vi "HEWH Filter All Temps.vi"(6 "Good Scan?":bool, 8 "error in (no error)":errorcluster, 11 "Pressure Adjusted in":T1) -> (0 "error out":errorcluster, 2 "TC Tree Array":dbl[](array[numeric]), 3 "Pressure Adjusted out":T1)   [LabVIEW 2023]
uses:
  Type Definitions/HEWH MW100 Data Cluster.ctl
  <vilib>/Analysis/NI_AALBase.lvlib
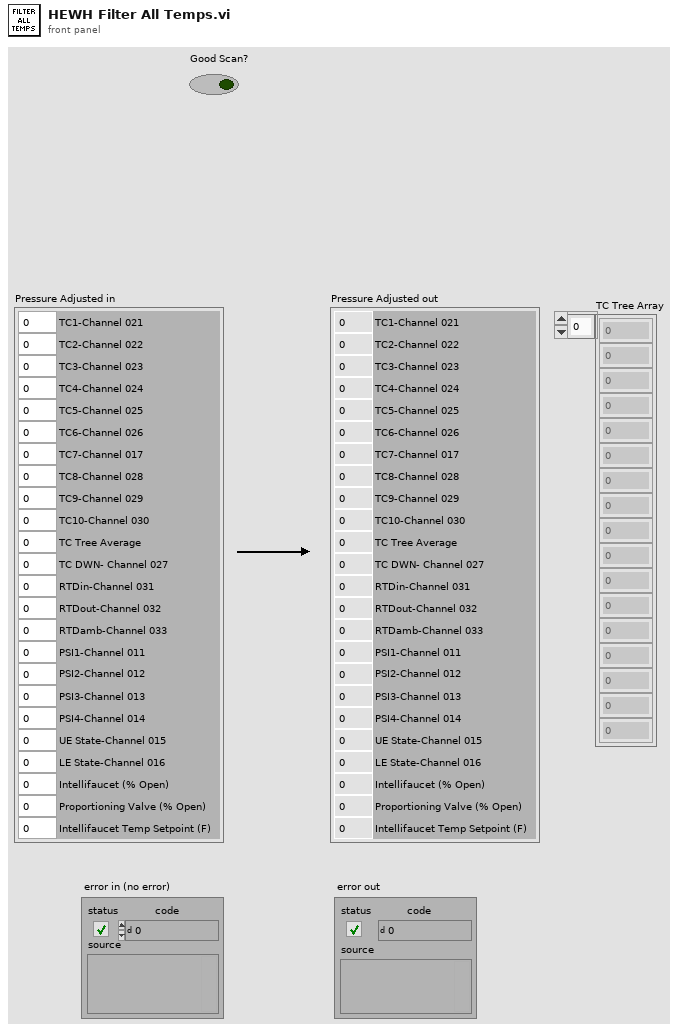
[diagram p1: front panel]
types:
  T1 = typedef "HEWH MW100 Data Cluster.ctl" = cluster{"TC1-Channel 021":dbl, "TC2-Channel 022":dbl, "TC3-Channel 023":dbl, "TC4-Channel 024":dbl, "TC5-Channel 025":dbl, "TC6-Channel 026":dbl, "TC7-Channel 017":dbl, "TC8-Channel 028":dbl, "TC9-Channel 029":dbl, "TC10-Channel 030":dbl, "TC Tree Average":dbl, "TC DWN- Channel 027":dbl, "RTDin-Channel 031":dbl, "RTDout-Channel 032":dbl, "RTDamb-Channel 033":dbl, "PSI1-Channel 011":dbl, "PSI2-Channel 012":dbl, "PSI3-Channel 013":dbl, "PSI4-Channel 014":dbl, "UE State-Channel 015":dbl, "LE State-Channel 016":dbl, "Intellifaucet (% Open)":dbl, "Proportioning Valve (% Open)":dbl, "Intellifaucet Temp Setpoint (F)":dbl}
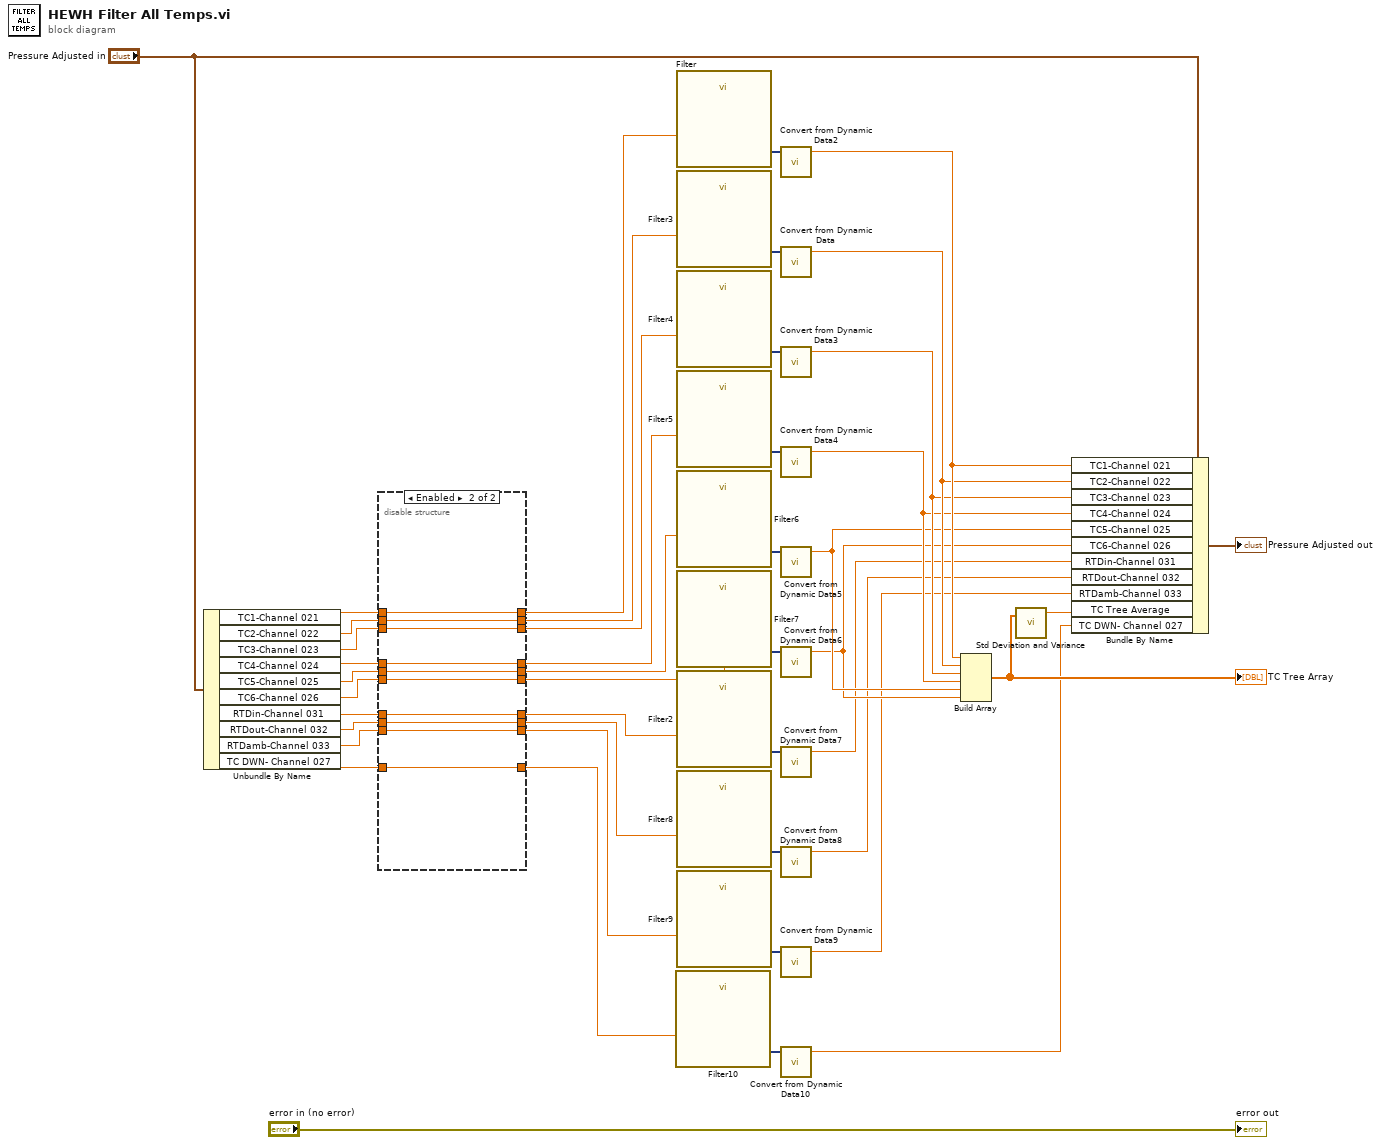
[diagram p0: block diagram]
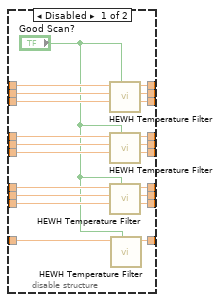
[diagram p2: hidden frame]
diagram:
  n1 = Unbundle By Name("Pressure Adjusted in") -> ("TC1-Channel 021"=w42:dbl, "TC2-Channel 022"=w41:dbl, "TC3-Channel 023"=w40:dbl, "TC4-Channel 024"=w39:dbl, "TC5-Channel 025"=w38:dbl, "TC6-Channel 026"=w37:dbl, "RTDin-Channel 031"=w36:dbl, "RTDout-Channel 032"=w35:dbl, "RTDamb-Channel 033"=w34:dbl, "TC DWN- Channel 027"=w5:dbl)
  n2 = disable-structure shown="Enabled" {
    disable-tunnel: w42 -> [w66 w76]
    disable-tunnel: w41 -> [w65 w75]
    disable-tunnel: w40 -> [w64 w74]
    disable-tunnel: w39 -> [w63 w73]
    disable-tunnel: w38 -> [w62 w72]
    disable-tunnel: w37 -> [w61 w71]
    disable-tunnel: w36 -> [w60 w70]
    disable-tunnel: w35 -> [w59 w69]
    disable-tunnel: w34 -> [w58 w68]
    disable-tunnel: [w57 w76] -> w33
    disable-tunnel: [w56 w74] -> w32
    disable-tunnel: [w55 w73] -> w31
    disable-tunnel: [w54 w72] -> w30
    disable-tunnel: [w53 w71] -> w29
    disable-tunnel: [w52 w70] -> w28
    disable-tunnel: [w51 w69] -> w27
    disable-tunnel: [w50 w68] -> w26
    disable-tunnel: [w49 w75] -> w14
    disable-tunnel: w5 -> [w48 w67]
    disable-tunnel: [w46 w67] -> w2
    frame Disabled {
      n3 = call "HEWH Temperature Filter.vi"("Good Scan?"="Good Scan?", "Temperature 3 Inlet"=w64, "Temperature 2 Inlet"=w65, "Temperature 1 Inlet"=w66) -> ("Temperature 3 Outlet"=w56:dbl, "Temperature 2 Outlet"=w49:dbl, "Temperature 1 Outlet"=w57:dbl)  [unwired: 5 in]
      n4 = call "HEWH Temperature Filter.vi"("Good Scan?"="Good Scan?", "Temperature 3 Inlet"=w61, "Temperature 2 Inlet"=w62, "Temperature 1 Inlet"=w63) -> ("Temperature 3 Outlet"=w53:dbl, "Temperature 2 Outlet"=w54:dbl, "Temperature 1 Outlet"=w55:dbl)  [unwired: 5 in]
      n5 = call "HEWH Temperature Filter.vi"("Good Scan?"="Good Scan?", "Temperature 3 Inlet"=w58, "Temperature 2 Inlet"=w59, "Temperature 1 Inlet"=w60) -> ("Temperature 3 Outlet"=w50:dbl, "Temperature 2 Outlet"=w51:dbl, "Temperature 1 Outlet"=w52:dbl)  [unwired: 5 in]
      n6 = call "HEWH Temperature Filter.vi"("Good Scan?"="Good Scan?", "Temperature 1 Inlet"=w48) -> ("Temperature 1 Outlet"=w46:dbl)  [unwired: 7 in, 2 out]
    }
    frame Enabled {
    }
  }
  n7 = call "Filter10"("Signal"=w2) -> ("Filtered Signal"=w4:dynamicdata)  [unwired: 9 in, 1 out]
  n8 = call "Filter"("Signal"=w33) -> ("Filtered Signal"=w25:dynamicdata)  [unwired: 9 in, 1 out]
  n9 = call "Filter3"("Signal"=w14) -> ("Filtered Signal"=w24:dynamicdata)  [unwired: 9 in, 1 out]
  n10 = call "Filter4"("Signal"=w32) -> ("Filtered Signal"=w23:dynamicdata)  [unwired: 9 in, 1 out]
  n11 = call "Filter5"("Signal"=w31) -> ("Filtered Signal"=w22:dynamicdata)  [unwired: 9 in, 1 out]
  n12 = call "Filter6"("Signal"=w30) -> ("Filtered Signal"=w21:dynamicdata)  [unwired: 9 in, 1 out]
  n13 = call "Filter7"("Signal"=w29) -> ("Filtered Signal"=w20:dynamicdata)  [unwired: 9 in, 1 out]
  n14 = call "Filter2"("Signal"=w28) -> ("Filtered Signal"=w19:dynamicdata)  [unwired: 9 in, 1 out]
  n15 = call "Filter8"("Signal"=w27) -> ("Filtered Signal"=w18:dynamicdata)  [unwired: 9 in, 1 out]
  n16 = call "Filter9"("Signal"=w26) -> ("Filtered Signal"=w17:dynamicdata)  [unwired: 9 in, 1 out]
  n17 = call "Convert from Dynamic Data2"("Dynamic Data Type"=w25) -> ("Scalar"=w15:dbl)  [unwired: 3 in]
  n18 = call "Convert from Dynamic Data"("Dynamic Data Type"=w24) -> ("Scalar"=w13:dbl)  [unwired: 3 in]
  n19 = call "Convert from Dynamic Data3"("Dynamic Data Type"=w23) -> ("Scalar"=w12:dbl)  [unwired: 3 in]
  n20 = call "Convert from Dynamic Data4"("Dynamic Data Type"=w22) -> ("Scalar"=w11:dbl)  [unwired: 3 in]
  n21 = call "Convert from Dynamic Data5"("Dynamic Data Type"=w21) -> ("Scalar"=w10:dbl)  [unwired: 3 in]
  n22 = call "Convert from Dynamic Data6"("Dynamic Data Type"=w20) -> ("Scalar"=w9:dbl)  [unwired: 3 in]
  n23 = call "Convert from Dynamic Data7"("Dynamic Data Type"=w19) -> ("Scalar"=w8:dbl)  [unwired: 3 in]
  n24 = call "Convert from Dynamic Data8"("Dynamic Data Type"=w18) -> ("Scalar"=w7:dbl)  [unwired: 3 in]
  n25 = call "Convert from Dynamic Data9"("Dynamic Data Type"=w17) -> ("Scalar"=w6:dbl)  [unwired: 3 in]
  n26 = call "Convert from Dynamic Data10"("Dynamic Data Type"=w4) -> ("Scalar"=w3:dbl)  [unwired: 3 in]
  n27 = Build Array(w15, w13, w12, w11, w10, w9) -> (w16:dbl[])
  "TC Tree Array" <- w16
  n28 = call <vilib>:"Std Deviation and Variance.vi"("X"=w16) -> ("mean"=w43:dbl)  [unwired: 1 in, 2 out]
  n29 = Bundle By Name(cluster="Pressure Adjusted in", "TC1-Channel 021"=w15, "TC2-Channel 022"=w13, "TC3-Channel 023"=w12, "TC4-Channel 024"=w11, "TC5-Channel 025"=w10, "TC6-Channel 026"=w9, "RTDin-Channel 031"=w8, "RTDout-Channel 032"=w7, "RTDamb-Channel 033"=w6, "TC Tree Average"=w43, "TC DWN- Channel 027"=w3) -> (→"Pressure Adjusted out":T1)
  "error out" <- "error in (no error)"
